vi "edit2.vi"(8 "error in (no error)":errorcluster, 11 "BaseSetting in":refnum<class "ProcessSetting.lvclass">) -> (0 "error out":errorcluster, 2 "cancelIsTrue out":bool, 3 "BaseSetting out":refnum<class "ProcessSetting.lvclass">)   [LabVIEW 2016]
uses:
  <vilib>/Utility/xml.llb/Write to XML File(string).vi
  Settings/Setting.lvclass
  ProcessSetting/ProcessSetting.lvclass
  D:/Code/ts_M1M3Support/Settings/Settings/Setting.lvclass
  Communicator/DataTypes/M1M3SALSettings.ctl
  Communicator/M1M3Communicator.lvlib
  Types/Settings/Base/SettingAlias.ctl
  Types/M1M3SupportTypes.lvlib
  Types/Settings/Base/SettingAliases.ctl
  Types/Settings/Base/RecommendedSettings.ctl
  Types/Settings/Base/BaseILCIdentitySettings.ctl
  Types/Settings/Base/BaseHPSettings.ctl
  Common_RT_HPILC/DataTypes/HPTimings.ctl
  Common_RT_HPILC/RTHPILC.lvlib
  Common_RT_ILC/DataTypes/ILCTimings.ctl
  Common_RT_ILC/RTILC.lvlib
  Types/Settings/Base/BaseILCSettings.ctl
panel:
  in  "SettingTab":T1(tab)
  in  "Aliases":T2
  in  "RecommendedSettings":T4
  in  "SALSettings":T5={"IPAddress"="127.0.0.1", "Port"=0, "StartupScript"="source /usr/ts_sal/setup.env && /usr/ts_sal/test/m1m3/cpp/src/SALPipe %d -1"}
  in  "ILCSettings":T6
  in  "HPSettings":T8
  in  "cancelIsTrue":bool
  out "String":string
  in  "saveIsTrue":bool
  in  "Listbox":i32(listbox)
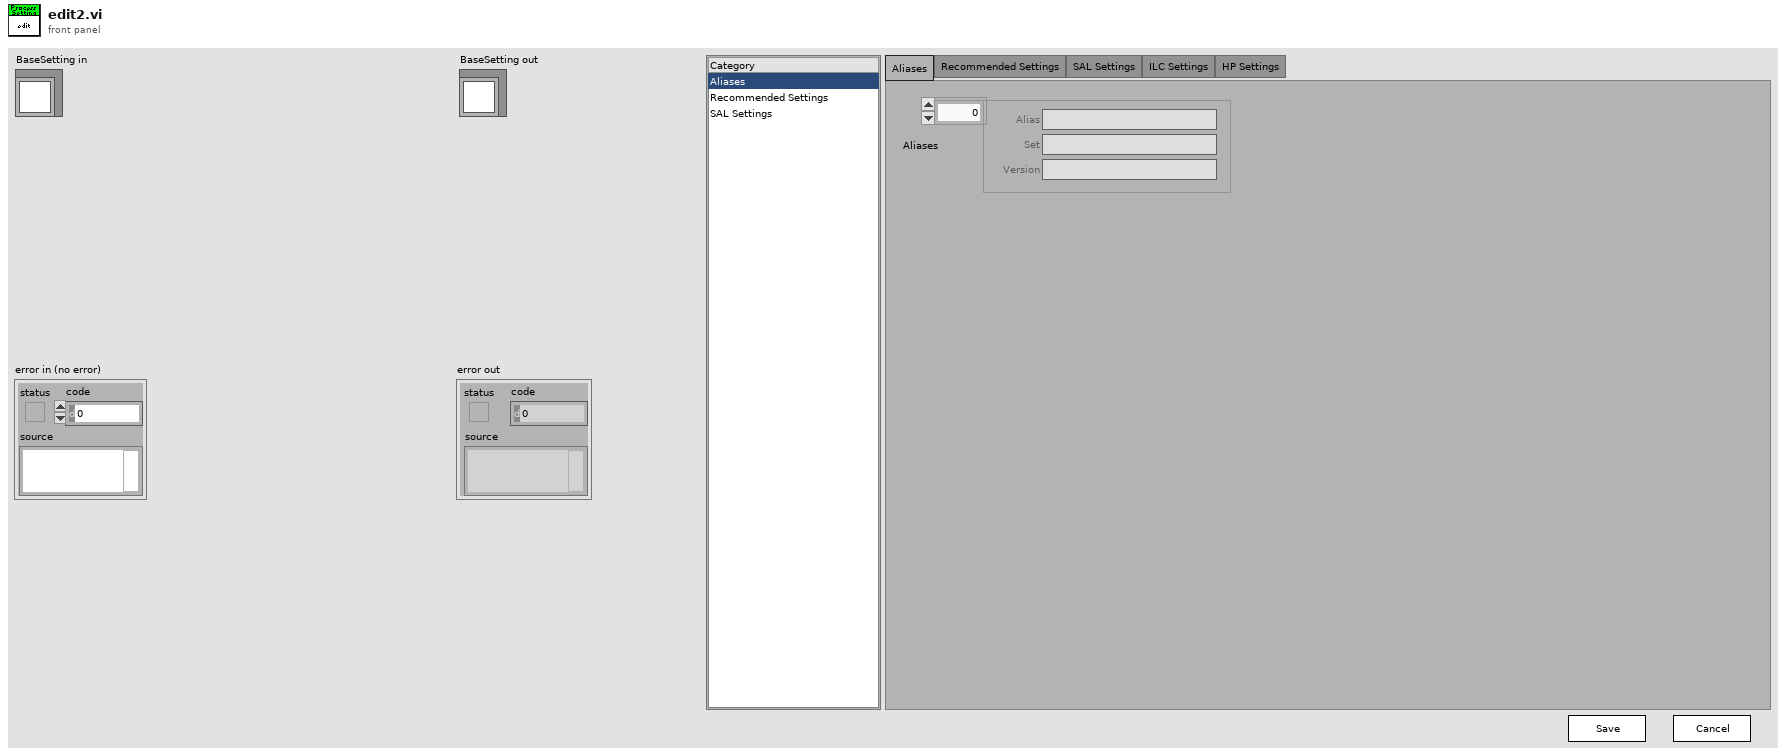
[diagram p1: front panel]
types:
  T1 = enum32{"Aliases", "Recommended Settings", "SAL Settings", "ILC Settings", "HP Settings"}
  T2 = typedef "M1M3SupportTypes.lvlib/SettingAliases.ctl" = cluster{"Aliases":T3[]}
  T3 = typedef "M1M3SupportTypes.lvlib/SettingAlias.ctl" = cluster{"Alias":string, "Set":string, "Version":string}
  T4 = typedef "M1M3SupportTypes.lvlib/RecommendedSettings.ctl" = cluster{"RecommendedSettings":string[]}
  T5 = typedef "M1M3Communicator.lvlib/M1M3SALSettings.ctl" = cluster{"IPAddress":string, "Port":u16, "StartupScript":string}
  T6 = typedef "M1M3SupportTypes.lvlib/BaseILCSettings.ctl" = cluster{"CommunicationTimings":T7}
  T7 = typedef "RTILC.lvlib/ILCTimings.ctl" = cluster{"ADCOffsetSensitivity":u32, "ADCScanRate":u32, "ILCMode":u32, "ReadCalibration":u32, "ReportServerID":u32, "ReportServerStatus":u32, "Reset":u32, "SetTemporaryAddress":u32}
  T8 = typedef "M1M3SupportTypes.lvlib/BaseHPSettings.ctl" = cluster{"Identification":T9[], "CommunicationTimings":T10}
  T9 = typedef "M1M3SupportTypes.lvlib/BaseILCIdentitySettings.ctl" = cluster{"Subnet":u8, "Address":u8, "ID":i16}
  T10 = typedef "RTHPILC.lvlib/HPTimings.ctl" = cluster{"BroadcastStepMotor":u32, "ForceAndStatus":u32, "FreezeSensorValues":u32, "StepMotor":u32}
  T11 = enum16{"open", "replace", "create", "open or create", "replace or create", "replace or create with confirmation"}
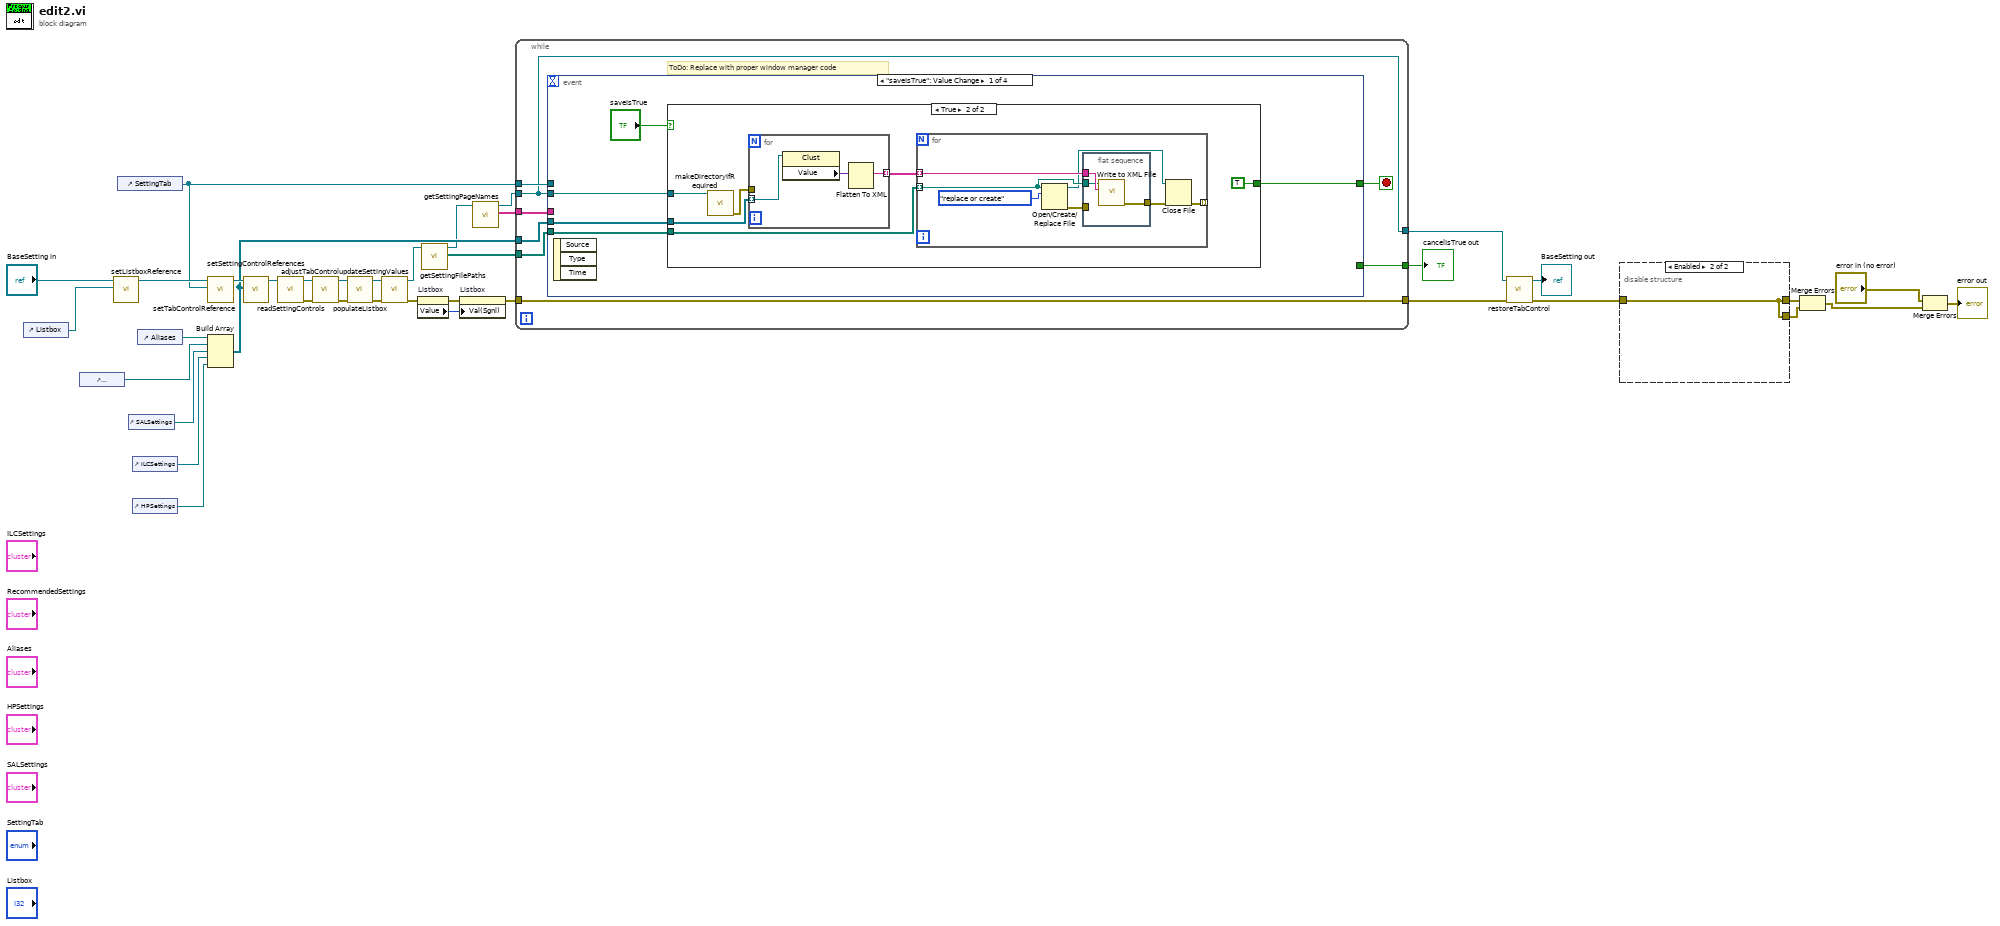
[diagram p0: block diagram]
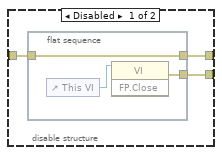
[diagram p2: hidden frame]
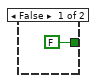
[diagram p3: hidden frame]
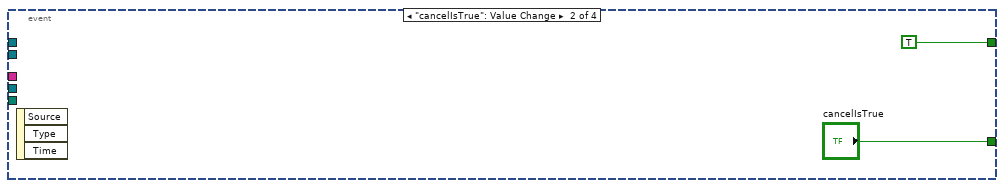
[diagram p4: hidden frame]
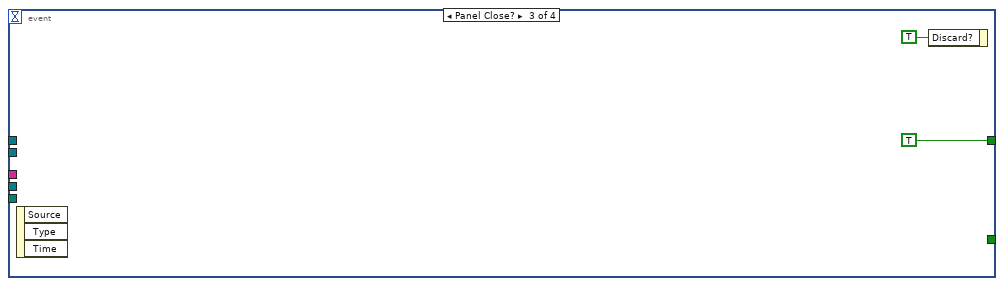
[diagram p5: hidden frame]
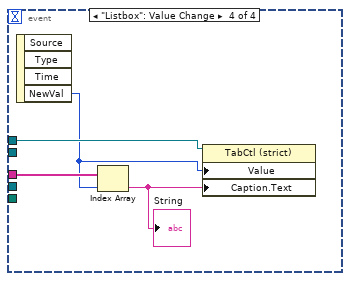
[diagram p6: hidden frame]
diagram:
  n1 = control-ref of="Listbox"() -> (w25:refnum<vi>)
  n2 = control-ref of="RecommendedSettings"() -> (w26:refnum<vi>)
  n3 = call "setListboxReference.vi"("ListboxReference"=w25, "Setting in"="BaseSetting in") -> ("Setting out"=w24:refnum<class "ProcessSetting.lvclass">)  [unwired: 9 in]
  n4 = control-ref of="SettingTab"() -> (w22:refnum<vi>)
  n5 = control-ref of="SALSettings"() -> (w28:refnum<vi>)
  n6 = control-ref of="ILCSettings"() -> (w1:refnum<vi>)
  n7 = control-ref of="HPSettings"() -> (w2:refnum<vi>)
  n8 = control-ref of="Aliases"() -> (w27:refnum<vi>)
  n9 = call "setTabControlReference.vi"("TabControlReference"=w22, "Setting in"=w24) -> ("Setting out"=w23:refnum<class "ProcessSetting.lvclass">)  [unwired: 9 in]
  n10 = Build Array(w27, w26, w28, w1, w2) -> (w21:refnum<vi>[])
  n11 = call "setSettingControlReferences.vi"("SettingControlReferences"=w21, "Setting in"=w23) -> ("Setting out"=w16:refnum<class "ProcessSetting.lvclass">)  [unwired: 9 in]
  n12 = call "readSettingControls.vi"("BaseSetting in"=w16) -> ("error out"=w11:errorcluster, "BaseSetting out"=w15:refnum<class "ProcessSetting.lvclass">)  [unwired: 9 in]
  n13 = call "adjustTabControl.vi"("error in (no error)"=w11, "BaseSetting in"=w15) -> ("error out"=w10:errorcluster, "BaseSetting out"=w14:refnum<class "ProcessSetting.lvclass">)  [unwired: 8 in]
  n14 = call "populateListbox.vi"("error in (no error)"=w10, "BaseSetting in"=w14) -> ("error out"=w9:errorcluster, "BaseSetting out"=w13:refnum<class "ProcessSetting.lvclass">)  [unwired: 8 in]
  n15 = call "updateSettingValues.vi"("error in (no error)"=w9, "BaseSetting in"=w13) -> ("error out"=w8:errorcluster, "BaseSetting out"=w12:refnum<class "ProcessSetting.lvclass">)  [unwired: 8 in]
  n16 = property on="Listbox" class="LstBox (strict)"(error in=w8) -> (error out=w36:errorcluster, "Value"=w37:i32)  [unwired: 1 in, 1 out]
  n17 = call "getSettingFilePaths.vi"("Setting in"=w12) -> ("SettingFilePaths"=w18:path[], "Setting out"=w20:refnum<class "ProcessSetting.lvclass">)  [unwired: 9 in]
  n18 = property on="Listbox" class="LstBox (strict)"(error in=w36, "Val(Sgnl)"=w37) -> (error out=w29:errorcluster)  [unwired: 1 in, 1 out]
  n19 = call "getSettingPageNames.vi"("Setting in"=w20) -> ("SettingPageNames"=w19:string[], "Setting out"=w17:refnum<class "ProcessSetting.lvclass">)  [unwired: 9 in]
  n20 = while {
    tunnel: w18 -> [w45]
    tunnel: w19 -> [w44]
    tunnel: w22 -> [w41]
    tunnel: w21 -> [w43]
    tunnel: [w38] -> w7
    tunnel: w17 -> [w38]
    tunnel: w29 -> [w40]
    tunnel: [w40] -> w4
    tunnel: [w39] -> w30
    stop <- w42 stop-if-true
    # "ToDo: Replace with proper window manager code"
    n21 = event shown="[0] \"saveIsTrue\": Value Change" {
      selector: _ -> [_ _ _ _]
      dyn-events: _ -> [_ _ _ _]
      timeout: _ -> [_ _ _ _]
      tunnel: [w46 TRUE TRUE _] -> w42
      tunnel: w45 -> [w50 _ _ _]
      tunnel: w44 -> [_ _ _ w77]
      tunnel: w41 -> [_ _ _ w78]
      tunnel: w43 -> [w49 _ _ _]
      tunnel: [_ "cancelIsTrue" _ _] -> w39
      tunnel: w38 -> [w48 _ _ _]
      event "saveIsTrue": Value Change {
        n22 = event-data() -> ()  [unwired: 1 in, 3 out]
        n23 = case shown="True" "saveIsTrue" {
          tunnel: w50 -> [_ w57]
          tunnel: w49 -> [_ w56]
          tunnel: w48 -> [_ w53]
          tunnel: [FALSE TRUE] -> w46
          frame False {
          }
          frame True {
            n24 = call "makeDirectoryIfRequired.vi"("BaseSetting in"=w53) -> ("error out"=w52:errorcluster)  [unwired: 9 in, 1 out]
            n25 = for {
              tunnel: w56 -> [w70] mode=indexing
              tunnel: [w68] -> w55 mode=indexing
              tunnel: w52 -> [_]
              n26 = property class="Clust"(reference=w70) -> ("Value"=w69:variant)  [unwired: 1 in, 2 out]
              n27 = Flatten To XML(anything=w69) -> (xml string=w68:string)
            }
            n28 = for {
              tunnel: w57 -> [w61] mode=indexing
              tunnel: w55 -> [w64] mode=indexing
              tunnel: [w58] -> _ mode=indexing
              n29 = Open/Create/Replace File(file path (use dialog)=w61, operation (0:open)=T11."replace or create") -> (refnum out=w60:refnum<file>, error out=w62:errorcluster)  [unwired: 4 in, 1 out]
              n30 = flat-sequence {
                tunnel: w64 -> [w67]
                tunnel: [w66] -> w59
                tunnel: w62 -> [_]
                tunnel: w61 -> [w65]
                frame #0 {
                  n31 = call-poly <vilib>:"Write to XML File.vi"("XML Input"=w67, "XML File Path"=w65) -> ("error out"=w66:errorcluster)  [unwired: 7 in, 2 out]
                }
              }
              n32 = Close File(refnum=w60, error in=w59) -> (error out=w58:errorcluster)  [unwired: 1 out]
            }
          }
        }
      }
      event "cancelIsTrue": Value Change {
        n33 = event-data() -> ()  [unwired: 1 in, 3 out]
      }
      event Panel Close? {
        n34 = event-data() -> ()  [unwired: 1 in, 3 out]
        n35 = event-data("Discard?"=TRUE) -> ()  [unwired: 1 in, 1 out]
      }
      event "Listbox": Value Change {
        n36 = event-data() -> ("NewVal"=w76:i32)  [unwired: 1 in, 3 out]
        n37 = Index Array(array=w77, index=w76) -> (element=w75:string)
        "String" <- w75
        n38 = property class="TabCtl (strict)"(reference=w78, "Value"=w76, "Caption.Text"=w75) -> ()  [unwired: 1 in, 2 out]
      }
    }
  }
  "cancelIsTrue out" <- w30
  n39 = call "restoreTabControl.vi"("error in (no error)"=w4, "BaseSetting in"=w7) -> ("error out"=w5:errorcluster, "BaseSetting out"=→"BaseSetting out":refnum<class "ProcessSetting.lvclass">)  [unwired: 8 in]
  n40 = disable-structure shown="Enabled" {
    disable-tunnel: [w81 w85] -> w33
    disable-tunnel: [w80 w85] -> w31
    disable-tunnel: w5 -> [w79 w85]
    frame Disabled {
      n41 = flat-sequence {
        tunnel: [w83] -> w81
        tunnel: [w82] -> w80
        tunnel: w79 -> [w82]
        frame #0 {
          n42 = control-ref of="This VI"() -> (w84:refnum<vi>)
          n43 = invoke class="VI" method="FP.Close"(reference=w84) -> (error out=w83:errorcluster)  [unwired: 2 in, 2 out]
        }
      }
    }
    frame Enabled {
    }
  }
  n44 = Merge Errors(w31, w33) -> (w32:errorcluster)
  n45 = Merge Errors("error in (no error)", w32) -> (→"error out":errorcluster)
